vi "Shooter Simulator Set Angle Motor.vi"(10 "Angle Motor Power":dbl) -> ()   [LabVIEW 2015]
uses:
  Shooter Simulator Globals.vi
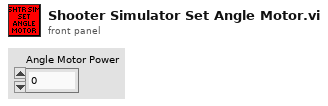
[diagram p1: front panel]
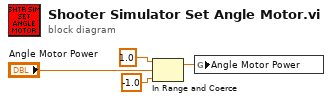
[diagram p0: block diagram]
diagram:
  n1 = In Range and Coerce(upper limit=1.0, x="Angle Motor Power", lower limit=-1.0) -> (coerced(x)=w1:dbl)  [unwired: 1 out]
  n2 = global write "Shooter Simulator Globals.vi" "Angle Motor Power"(w1) -> ()
